vi "Single Count Test.vi"() -> ()   [LabVIEW 2012]
panel:
  out "Total":i64
  out "Total":i64
  out "Coincidence Count SS1":i64
  in  "Window Offset 1 (ns)":i32
  in  "Window Length 1 (ns)":i32
  in  "Stop Delay 1 (ns)":i16
  in  "Start-Stop1 Multyplex":T1
  in  "Start Measurement":bool
  out "Single Count Channel4":i64
  out "Single Count Channel3":i64
  out "Single Count Channel2":i64
  out "Single Count Channel1":i64
  out "Exposition time (ms)":i64
  out "Measurement index":i64
  out "Start OK":bool
  in  "Exit":bool
  in  "Single Count Enable":T2
  in  "Channel4 Pulse Front":string
  in  "Channel4 Threshold Voltage (mV)":i32
  in  "Channel3 Pulse Front":string
  in  "Channel3 Threshold Voltage (mV)":i32
  in  "Channel2 Pulse Front":string
  in  "Channel2 Threshold Voltage (mV)":i32
  in  "Channel1 Pulse Front":string(combo)
  in  "Channel1 Threshold Voltage (mV)":i32 min=0 max=5000 step=10
  in  "Exposition Time (ms)":i64
  # "Start from 0\n0 -> Channel1\n1 -> Channel2"
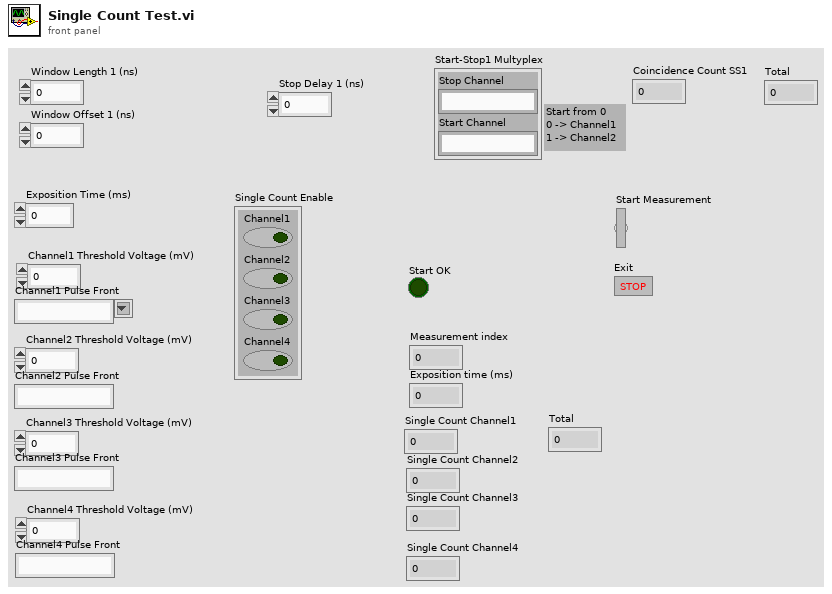
[diagram p1: front panel]
types:
  T1 = cluster{"Stop Channel":string, "Start Channel":string}
  T2 = cluster{"Channel1":bool, "Channel2":bool, "Channel3":bool, "Channel4":bool}
  T3 = cluster{"[0]":i64, "Channel1 Threshold Voltage (mV)":i32, "Channel1 Pulse Front":string, "Channel2 Threshold Voltage (mV)":i32, "Channel2 Pulse Front":string, "Channel3 Threshold Voltage (mV)":i32, "Channel3 Pulse Front ":string, "Channel4 Threshold Voltage (mV)":i32, "Channel4 Pulse Front ":string, "Single Count Enable":cluster{"Channel1":bool, "Channel2":bool, "Channel3":bool, "Channel4":bool}, "Single Count Max":i32, "Sum Count Enable":cluster{"Channel1":bool, "Channel2":bool, "Channel3":bool, "Channel4":bool}, "Sum Count Max":i32, "Start-Stop1 Multyplex":cluster{"Stop Channel":string, "Start Channel":string}, "Stop Delay 1 (ns)":i16, "Window Length 1 (ns)":i32, "Window Offset 1 (ns) ":i32, "Conditional Correlation 1":string, "Histogram Bin 1":string, "Histogram Start 1 (ns) ":i32, "Start-Stop2 Multyplex ":cluster{"Stop Channel":string, "Start Channel":string}, "Stop Delay 2 (ns)":i16, "Window Length 2 (ns) ":i32, "Window Offset 2 (ns) ":i32, "Conditional Correlation 2":string, "Histogram Bin 2":string, "Histogram Start 2 (ns)  ":i32, "Start-Stop3 Multyplex":cluster{"Stop Channel":string, "Start Channel":string}, "Stop Delay 3 (ns)":i16, "Window Length 3 (ns) ":i32, "Window Offset 3 (ns) ":i32, "Conditional Correlation 3":string, "Histogram Bin 3":string, "Histogram Start 3 (ns) ":i32, "Start-Stop4 Multyplex":cluster{"Stop Channel":string, "Start Channel":string}, "Stop Delay 4 (ns)":i16, "Window Length 4 (ns)  ":i32, "Window Offset 4 (ns) ":i32, "Conditional Correlation 4":string, "Histogram Bin 4":string, "Histogram Start 4 (ns)  ":i32, "Coincidence Count Enable":cluster{"Start-Stop1":bool, "Start-Stop2":bool, "Start-Stop3":bool, "Start-Stop4":bool}, "Coincidence Count Max":i32, "Coincidence Sum Enable":cluster{"Start-Stop1":bool, "Start-Stop2":bool, "Start-Stop3":bool, "Start-Stop4":bool}, "Coincidence Sum Max":i32, "Output Channel Enable":cluster{"Channel1":bool, "Channel2":bool, "Channel3":bool, "Channel4":bool}, "Output Channel Inversion":cluster{"Channel1":bool, "Channel2":bool, "Channel3":bool, "Channel4":bool, "Output":bool}}
  T4 = cluster{"Going":bool, "Iinterrupted":bool, "Timer stop":bool, "Single count stop Ch1":bool, "Single count stop Ch2":bool, "Single count stop Ch3":bool, "Single count stop Ch4":bool, "Sum count stop":bool, "Coincidence count stop SS1":bool, "Coincidence count stop SS2":bool, "Coincidence count stop SS3":bool, "Coincidence count stop SS4":bool, "Coincidence sum count stop":bool, "Reserved":bool, "Correlator is not initialised":bool, "Internal error":bool}
  T5 = cluster{"Measurement index":i64, "Exposition time (ms)":i64, "Single Count Channel1":i64, "Single Count Channel2":i64, "Single Count Channel3":i64, "Single Count Channel4":i64, "Sum Single Count":i64, "Coincidence Count SS1":i64, "Coincidence Count SS2":i64, "Coincidence Count SS4":i64, "Coincidence Count SS5":i64, "Sum Coincidence Count":i64}
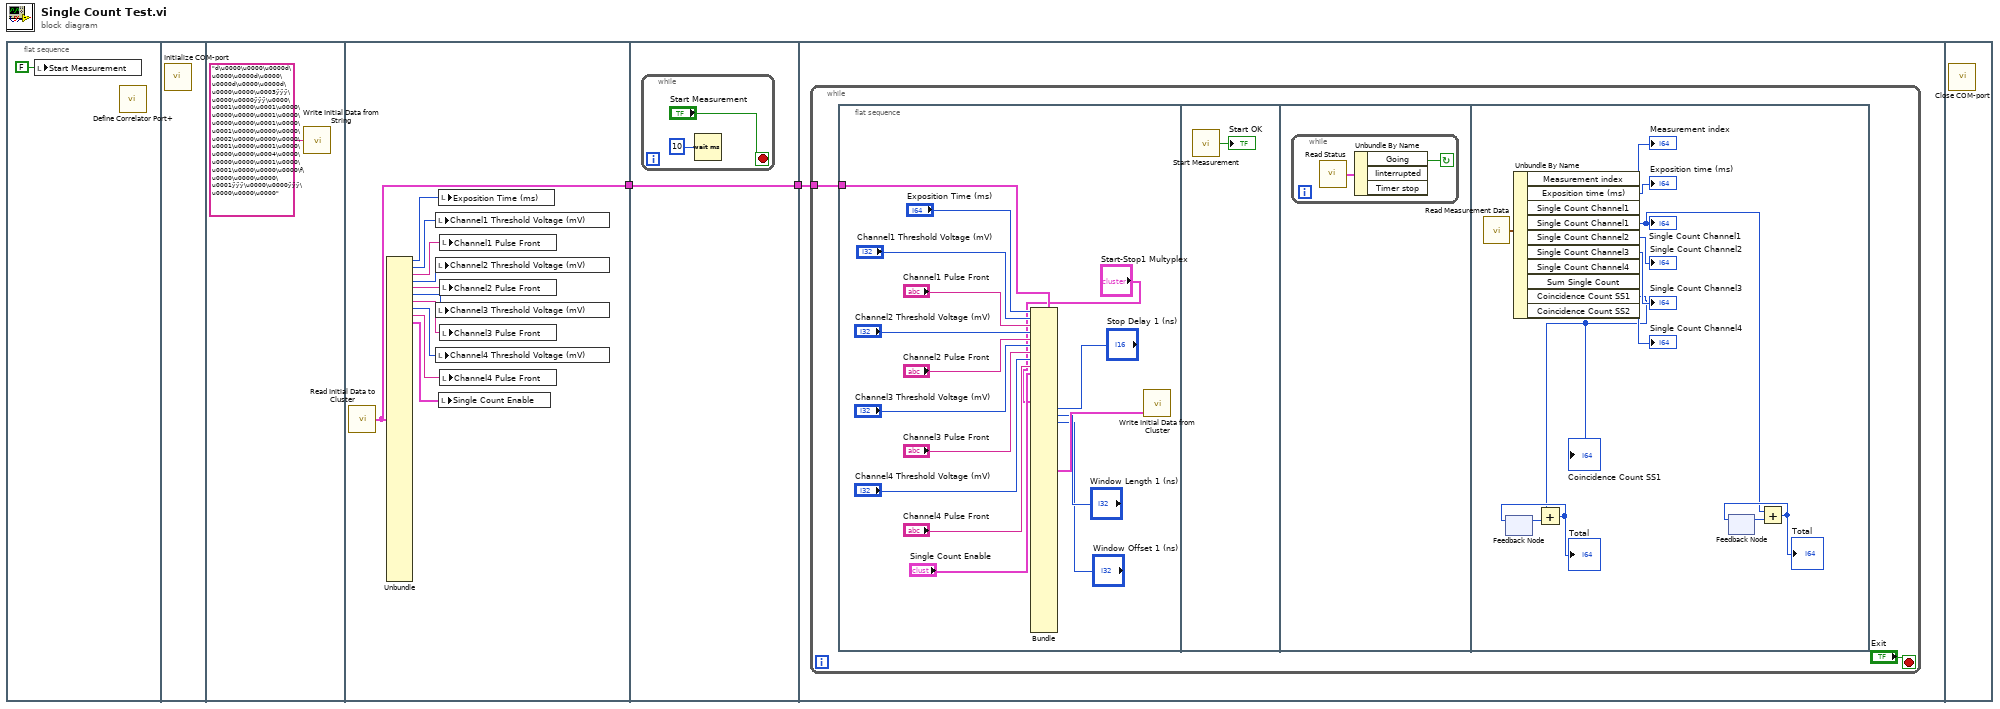
[diagram p0: block diagram]
diagram:
  n1 = flat-sequence {
    tunnel: [w15] -> w2
    tunnel: w2 -> [w16]
    tunnel: [w16] -> w1
    tunnel: w1 -> [w19]
    frame #0 {
      n2 = local write "Start Measurement"(FALSE ("Start Measurement")) -> ()
      n3 = call "Define Correlator Port+.vi"() -> ()  [unwired: 3 in]
    }
    frame #1 {
      n4 = call "Initialize COM-port.vi"() -> ()  [unwired: 4 in]
    }
    frame #2 {
      n5 = call "Write Initial Data from String.vi"("Data"="d\u0000\u0000\u0000d\u0000\u0000d\u0000\u0000d\u0000\u0000d\u0000\u0000\u0003ÿÿÿ\u0000\u0000ÿÿÿ\u0000\u0001\u0000\u0001\u0000\u0000\u0000\u0001\u0000\u0000\u0000\u0001\u0000\u0001\u0000\u0000\u0000\u0002\u0000\u0000\u0000\u0001\u0000\u0001\u0000\u0000\u0000\u0004\u0000\u0000\u0000\u0001\u0000\u0001\u0000\u0000\u0000\f\u0000\u0000\u0000\u0001ÿÿÿ\u0000\u0000ÿÿÿ\u0000\u0000\u0000") -> ()  [unwired: 1 out]
    }
    frame #3 {
      n6 = call "Read Initial Data to Cluster.vi"() -> ("Correlator Initial Data 2"=w15:T3)  [unwired: 2 in]
      n7 = Unbundle(w15) -> ("[0]"=w14:i64, "Channel1 Threshold Voltage (mV)"=w13:i32, "Channel1 Pulse Front"=w12:string, "Channel2 Threshold Voltage (mV)"=w11:i32, "Channel2 Pulse Front"=w10:string, "Channel3 Threshold Voltage (mV)"=w9:i32, "Channel3 Pulse Front"=w8:string, "Channel4 Threshold Voltage (mV)"=w7:i32, "Channel4 Pulse Front"=w6:string, "Single Count Enable"=w5:T2)  [unwired: 37 out]
      n8 = local write "Channel1 Threshold Voltage (mV)"(w13) -> ()
      n9 = local write "Channel2 Threshold Voltage (mV)"(w11) -> ()
      n10 = local write "Channel3 Threshold Voltage (mV)"(w9) -> ()
      n11 = local write "Channel4 Threshold Voltage (mV)"(w7) -> ()
      n12 = local write "Exposition Time (ms)"(w14) -> ()
      n13 = local write "Single Count Enable"(w5) -> ()
      n14 = local write "Channel1 Pulse Front"(w12) -> ()
      n15 = local write "Channel2 Pulse Front"(w10) -> ()
      n16 = local write "Channel3 Pulse Front"(w8) -> ()
      n17 = local write "Channel4 Pulse Front"(w6) -> ()
    }
    frame #4 {
      n18 = while {
        stop <- "Start Measurement" stop-if-true
        n19 = Wait (ms)(milliseconds to wait=u32 10) -> ()  [unwired: 1 out]
      }
    }
    frame #5 {
      n20 = while {
        tunnel: w19 -> [w20]
        stop <- "Exit" stop-if-true
        n21 = flat-sequence {
          tunnel: w20 -> [w29]
          frame #0 {
            n22 = Bundle(cluster=w29, "[0]"="Exposition Time (ms)", "Channel1 Threshold Voltage (mV)"="Channel1 Threshold Voltage (mV)", "Channel1 Pulse Front"="Channel1 Pulse Front", "Channel2 Threshold Voltage (mV)"="Channel2 Threshold Voltage (mV)", "Channel2 Pulse Front"="Channel2 Pulse Front", "Channel3 Threshold Voltage (mV)"="Channel3 Threshold Voltage (mV)", "Channel3 Pulse Front"="Channel3 Pulse Front", "Channel4 Threshold Voltage (mV)"="Channel4 Threshold Voltage (mV)", "Channel4 Pulse Front"="Channel4 Pulse Front", "Single Count Enable"="Single Count Enable", "Start-Stop1 Multyplex"="Start-Stop1 Multyplex", "Stop Delay 1 (ns)"="Stop Delay 1 (ns)", "Window Length 1 (ns)"="Window Length 1 (ns)", "Window Offset 1 (ns)"="Window Offset 1 (ns)") -> (w37:T3)  [unwired: 33 in]
            n23 = call "Write Initial Data from Cluster.vi"("Correlator Initial Data"=w37) -> ()  [unwired: 2 in, 1 out]
          }
          frame #1 {
            n24 = call "Start Measurement.vi"() -> ("Start OK"=→"Start OK":bool)  [unwired: 2 in]
          }
          frame #2 {
            n25 = while {
              stop <- w39 continue-if-true
              n26 = call "Read Status.vi"() -> ("Status Data"=w40:T4)  [unwired: 2 in]
              n27 = Unbundle By Name(w40) -> ("Going"=w39:bool)  [unwired: 2 out]
            }
          }
          frame #3 {
            n28 = call "Read Measurement Data.vi"() -> ("Measurement Data"=w52:T5)  [unwired: 3 in]
            n29 = feedback #1() -> (w46:i64)  [unwired: 1 in]
            n30 = Unbundle By Name(w52) -> ("Measurement index"=→"Measurement index":i64, "Exposition time (ms)"=→"Exposition time (ms)":i64, "Single Count Channel1"=w41:i64, "Single Count Channel2"=→"Single Count Channel2":i64, "Single Count Channel3"=→"Single Count Channel3":i64, "Single Count Channel4"=→"Single Count Channel4":i64, "Coincidence Count SS1"=w44:i64)  [unwired: 3 out]
            "Single Count Channel1" <- w41
            "Coincidence Count SS1" <- w44
            n31 = Add(x=w44, y=w46) -> (x+y=w45:i64)
            "Total" <- w45
            n32 = feedback-in #1(w45) -> ()
            n33 = feedback #2() -> (w43:i64)  [unwired: 1 in]
            n34 = Add(x=w41, y=w43) -> (x+y=w42:i64)
            "Total" <- w42
            n35 = feedback-in #2(w42) -> ()
          }
        }
      }
    }
    frame #6 {
      n36 = call "Close COM-port.vi"() -> ()  [unwired: 4 in]
    }
  }
